vi "database1查询.vi"(6 "时间2":string, 7 "error in (no error)":errorcluster, 8 "table":string, 9 "时间1":string, 10 "database":string="database1.mdb") -> (0 "error out":errorcluster, 2 "data":string[][](table), 3 "recordset data":variant[][](array[variant]))   [LabVIEW 2016, in "数据传输系统.lvlib"]
uses:
  <vilib>/Utility/sysdir.llb/System Directory Type.ctl
  <vilib>/addons/database/Connection.llb/DB Tools Open Connec (String).vi
  <vilib>/addons/database/Connection.llb/Conn Execute.vi
  <vilib>/addons/database/Recordset.llb/Rec Fetch Recordset Data (R).vi
  <vilib>/addons/database/Recordset.llb/Rec Destroy - Connection.vi
  <vilib>/addons/database/_DB Variant To Data/Database Variant To Data.xnode
  <vilib>/addons/database/NI_Database_API.lvlib
panel:
  out "SQL query":string
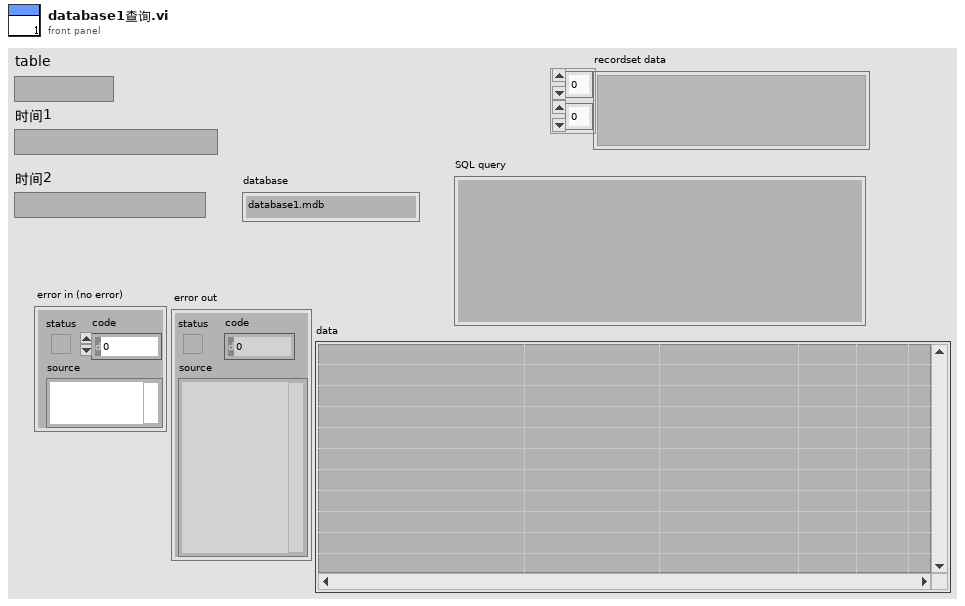
[diagram p1: front panel]
types:
  T1 = typedef "System Directory Type.ctl" = i32
  T2 = typedef "NI_Database_API.lvlib/Conn ObjectReference.ctl" = refnum<k1>
  T3 = typedef "NI_Database_API.lvlib/Rec ObjectReference.ctl" = refnum<k1>
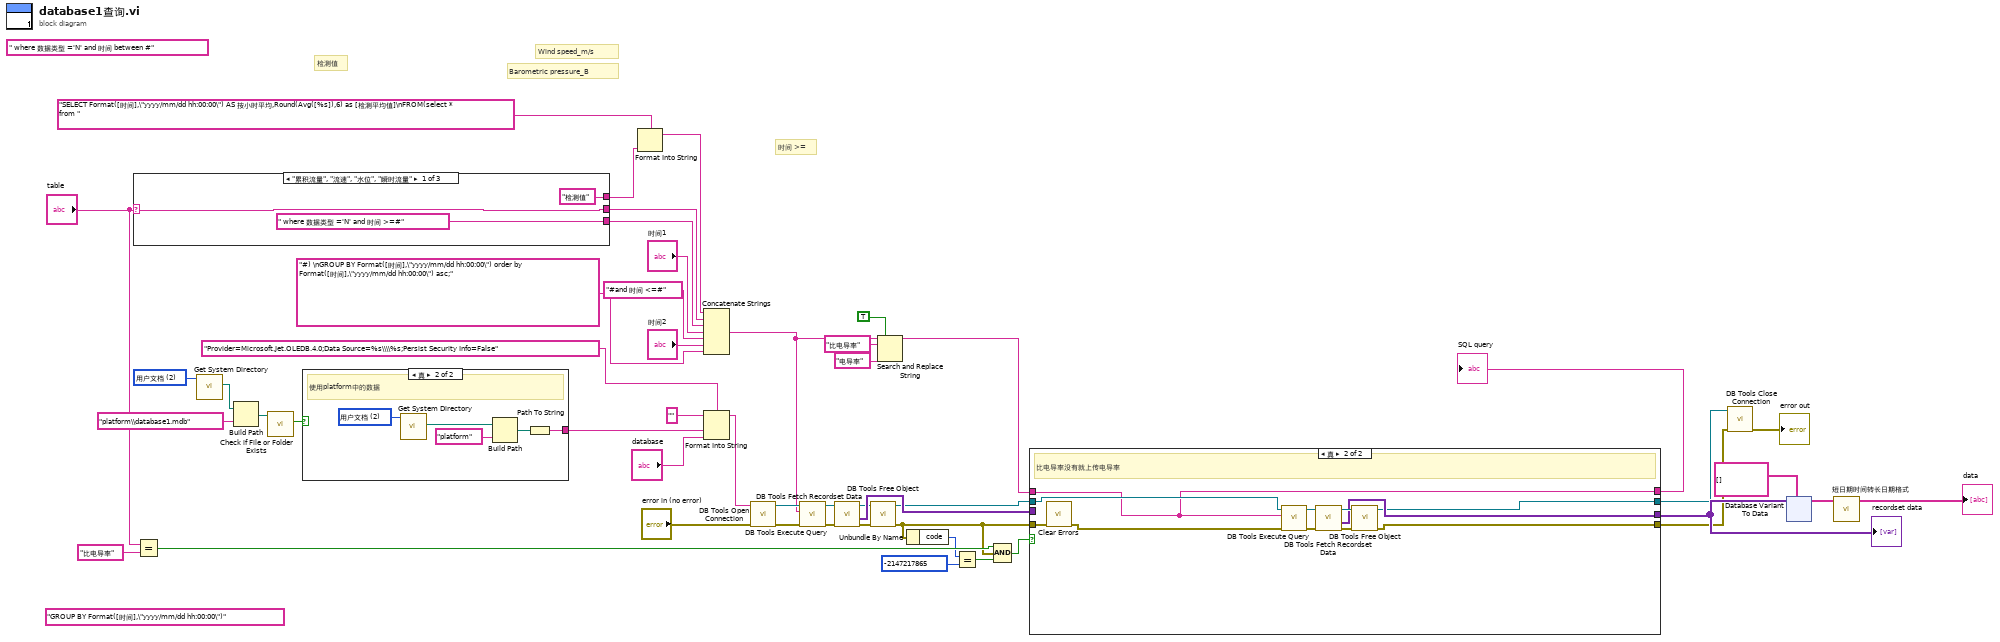
[diagram p0: block diagram]
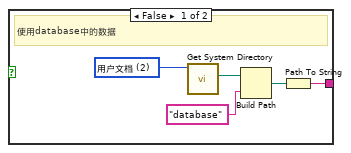
[diagram p3: hidden frame]
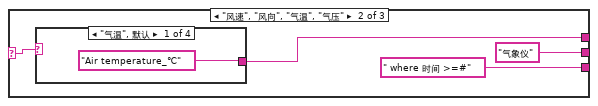
[diagram p4: hidden frame]
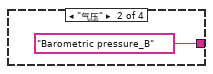
[diagram p5: hidden frame]
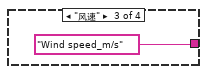
[diagram p6: hidden frame]
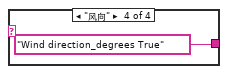
[diagram p7: hidden frame]
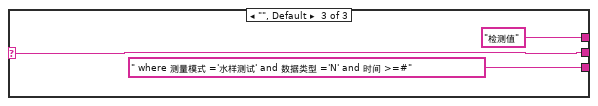
[diagram p8: hidden frame]
diagram:
  (unwired) " where 数据类型 ='N' and 时间 between #"
  w34 = T1 2 items=["用户目录"=0, "用户桌面"=1, "用户文档"=2, "用户应用程序数据"=3, "用户设置"=4, "用户临时目录"=5, "公共文档"=6, "公共应用程序数据"=7, "公共设置"=8, "公共缓存"=13, "系统核心库"=9, "系统安装库"=10, "应用程序文件"=11, "启动盘根目录"=12] ("system directory type")
  (unwired) "GROUP BY Format([时间],\"yyyy/mm/dd hh:00:00\")"
  # "时间 >="
  # "Wind speed_m/s"
  # "检测值"
  # "Barometric pressure_B"
  n1 = case shown="\"累积流量\", \"流速\", \"水位\", \"瞬时流量\"" "table" {
    selector: "table" -> [w51 w54 w62]
    tunnel: [" where 数据类型 ='N' and 时间 >=#" " where 时间 >=#" " where 测量模式 ='水样测试' and 数据类型 ='N' and 时间 >=#"] -> w38
    tunnel: ["检测值" w53 "检测值"] -> w4
    tunnel: [w51 "气象仪" w62] -> w2
    frame "累积流量", "流速", "水位", "瞬时流量" {
    }
    frame "风速", "风向", "气温", "气压" {
      n2 = case shown="\"气温\", 默认" w54 {
        tunnel: ["Air temperature_℃" "Barometric pressure_B" "Wind speed_m/s" "Wind direction_degrees True"] -> w53
        frame "气温", Default {
        }
        frame "气压" {
        }
        frame "风速" {
        }
        frame "风向" {
        }
      }
    }
    frame "", Default {
    }
  }
  n3 = Equal?(x="table", y="比电导率") -> (x = y?=w22:bool)
  n4 = call <vilib>:"Get System Directory.vi"("system directory type"=w34) -> ("system directory"=w35:path)  [unwired: 10 in]
  n5 = Build Path(base path=w35, name or relative path="platform\\database1.mdb" ("condition")) -> (appended path=w33:path)
  n6 = call <vilib>:"Check if File or Folder Exists.vi"("path"=w33) -> ("file or folder exists?"=w31:bool)  [unwired: 8 in, 2 out]
  n7 = case shown="真" w31 {
    tunnel: [w64 w69] -> w30
    frame False {
      w67 = T1 2 items=["用户目录"=0, "用户桌面"=1, "用户文档"=2, "用户应用程序数据"=3, "用户设置"=4, "用户临时目录"=5, "公共文档"=6, "公共应用程序数据"=7, "公共设置"=8, "公共缓存"=13, "系统核心库"=9, "系统安装库"=10, "应用程序文件"=11, "启动盘根目录"=12] ("system directory type")
      # "使用database中的数据"
      n8 = call <vilib>:"Get System Directory.vi"("system directory type"=w67) -> ("system directory"=w66:path)  [unwired: 10 in]
      n9 = Build Path(base path=w66, name or relative path="database" ("condition")) -> (appended path=w68:path)
      n10 = Path To String(path=w68) -> (string=w64:string)
    }
    frame True {
      w73 = T1 2 items=["用户目录"=0, "用户桌面"=1, "用户文档"=2, "用户应用程序数据"=3, "用户设置"=4, "用户临时目录"=5, "公共文档"=6, "公共应用程序数据"=7, "公共设置"=8, "公共缓存"=13, "系统核心库"=9, "系统安装库"=10, "应用程序文件"=11, "启动盘根目录"=12] ("system directory type")
      # "使用platform中的数据"
      n11 = call <vilib>:"Get System Directory.vi"("system directory type"=w73) -> ("system directory"=w72:path)  [unwired: 10 in]
      n12 = Build Path(base path=w72, name or relative path="platform" ("condition")) -> (appended path=w70:path)
      n13 = Path To String(path=w70) -> (string=w69:string)
    }
  }
  n14 = Format Into String(format string="SELECT Format([时间],\"yyyy/mm/dd hh:00:00\") AS 按小时平均,Round(Avg([%s]),6) as [检测平均值]\nFROM(select * from ", w4) -> (resulting string=w1:string)  [unwired: 2 in, 1 out]
  n15 = Concatenate Strings(w1, w2, w38, "时间1", "#and 时间 <=#", "时间2", "#) \nGROUP BY Format([时间],\"yyyy/mm/dd hh:00:00\") order by Format([时间],\"yyyy/mm/dd hh:00:00\") asc;" ("字符串")) -> (w12:string)
  n16 = Format Into String(format string="Provider=Microsoft.Jet.OLEDB.4.0;Data Source=%s\\\\%s;Persist Security Info=False" ("格式字符串"), initial string="" ("初始字符串"), w30, "database") -> (resulting string=w28:string)  [unwired: 1 in, 1 out]
  n17 = call-poly <vilib>:"DB Tools Open Connection.vi"("error in (no error)"="error in (no error)", "connection information"=w28) -> ("error out"=w46:errorcluster, "connection reference"=w24:T2)  [unwired: 6 in]
  n18 = call-poly <vilib>:"DB Tools Execute Query.vi"("error in (no error)"=w46, "SQL query"=w12, "connection reference"=w24) -> ("error out"=w20:errorcluster, "recordset reference"=w25:T3)  [unwired: 5 in]
  n19 = call-poly <vilib>:"DB Tools Fetch Recordset Data.vi"("error in (no error)"=w20, "recordset reference"=w25) -> ("error out"=w47:errorcluster, "recordset data"=w26:variant[][], "recordset reference out"=w21:T3)  [unwired: 3 in]
  n20 = call-poly <vilib>:"DB Tools Free Object.vi"("error in (no error)"=w47, "recordset reference"=w21) -> ("error out"=w14:errorcluster, "connection reference"=w18:T2)  [unwired: 8 in]
  n21 = Search and Replace String(replace all?=TRUE ("替换全部？(F)"), input string=w12, search string="比电导率" ("搜索字符串"), replace string="电导率" ("替换字符串(\"\")")) -> (result string=w9:string)  [unwired: 4 in, 3 out]
  n22 = Unbundle By Name(w14) -> ("code"=w16:i32)
  n23 = Equal?(x=w16, y=-2147217865 ("code")) -> (x = y?=w13:bool)
  n24 = Compound Arithmetic op=AND ("复合运算")(w22, w14, w13) -> (w27:bool)
  n25 = case shown="真" w27 {
    tunnel: w9 -> [w74 w78]
    tunnel: w18 -> [w75 w83]
    tunnel: [w75 w79] -> w17
    tunnel: [w77 w81] -> w19
    tunnel: w26 -> [w77 _]
    tunnel: w14 -> [w76 w88]
    tunnel: [w76 w80] -> w6
    tunnel: [w74 w78] -> w7
    frame False {
    }
    frame True {
      # "比电导率没有就上传电导率"
      n26 = call <vilib>:"Clear Errors.vi"("error in (no error)"=w88) -> ("error out"=w82:errorcluster)  [unwired: 5 in, 1 out]
      n27 = call-poly <vilib>:"DB Tools Execute Query.vi"("error in (no error)"=w82, "SQL query"=w78, "connection reference"=w83) -> ("error out"=w84:errorcluster, "recordset reference"=w86:T3)  [unwired: 5 in]
      n28 = call-poly <vilib>:"DB Tools Fetch Recordset Data.vi"("error in (no error)"=w84, "recordset reference"=w86) -> ("error out"=w87:errorcluster, "recordset data"=w81:variant[][], "recordset reference out"=w85:T3)  [unwired: 3 in]
      n29 = call-poly <vilib>:"DB Tools Free Object.vi"("error in (no error)"=w87, "recordset reference"=w85) -> ("error out"=w80:errorcluster, "connection reference"=w79:T2)  [unwired: 8 in]
    }
  }
  "SQL query" <- w7
  "recordset data" <- w19
  n30 = call <vilib>:"DB Tools Close Connection.vi"("error in (no error)"=w6, "connection reference"=w17) -> ("error out"=→"error out":errorcluster)  [unwired: 5 in]
  n31 = xnode "Database Variant To Data"("database variant"=w19, "type"=string[][] []) -> ("data"=w40:string[][])  [unwired: 1 in, 1 out]
  n32 = call "短日期时间转长日期格式.vi"("data"=w40) -> ("输出数组"=→"data":string[][])  [unwired: 10 in]
